vi "To More Specific Type (NULL).vi"(8 "error in (no error)":errorcluster, 11 "JSON Datatype in":refnum<class "JSON Null.lvclass">) -> (0 "error out":errorcluster, 3 "JSON Null out":refnum<class "JSON Null.lvclass">)   [LabVIEW 2016, in "LVJSON.lvlib" / "JSON Helper.lvclass"]
doc: "Casts a JSON instance to the given JSON type"
uses:
  JSON Helper.lvclass
  JSON Datatype/JSON Null.lvclass
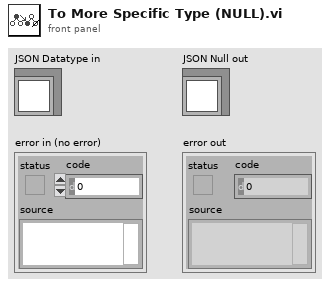
[diagram p1: front panel]
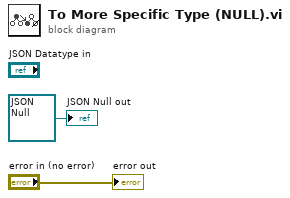
[diagram p0: block diagram]
diagram:
  "error out" <- "error in (no error)"
  "JSON Null out" <- refnum<class "JSON Null.lvclass"> refnum ("JSON Datatype out")
